vi "Finish.vi"   [LabVIEW 2016]
doc: "This VI is called just before exiting. It is expected to close I/O refnum, save collected data, etc."
uses:
  Climb/Climb Globals.vi
  Drive/Drive Globals.vi
  Intake/Intake Globals.vi
  Rotation/Rotation Globals.vi
  <vilib>/Rock Robotics/WPI/Utilities/WPI_GetSetVariantRefNum.vi
types:
  T1 = typedef "WPI_MotorControlDeviceRef.ctl" = cluster{"DeviceStatus":errorcluster, "Type":T2, "PWM":cluster{"PWM Channel":T3, "DeadBand":T4}, "CAN":cluster{"Device Number":u8, "SetOutput VI Ref":variant, "GetOutput VI Ref":variant, "Enable VI Ref":variant, "Disable VI Ref":variant, "Data":variant}, "Invert":bool}
  T2 = typedef "WPI_MotorControlType.ctl" = enum16{"PWM", "CAN"}
  T3 = typedef "FPGA_DIOPWMChannel.ctl" = enum8{"PWM 0", "PWM 1", "PWM 2", "PWM 3", "PWM 4", "PWM 5", "PWM 6", "PWM 7", "PWM 8", "PWM 9", "PWM MXP 0", "PWM MXP 1", "PWM MXP 2", "PWM MXP 3", "PWM MXP 4", "PWM MXP 5", "PWM MXP 6", "PWM MXP 7", "PWM MXP 8", "PWM MXP 9", "Invalid"}
  T4 = typedef "WPI_PWMDeadband.ctl" = cluster{"Name":string, "maxPositivePwm":i32, "minPositivePwm":i32, "centerPwm":i32, "maxNegativePwm":i32, "minNegativePwm":i32, "angularRange":u16}
  T5 = typedef "WPI_JoystickDevRef.ctl" = cluster{"Device":T6}
  T6 = typedef "WPI_JoystickDeviceEnum.ctl" = enum16{"USB 0", "USB 1", "USB 2", "USB 3", "USB 4", "USB 5"}
  T7 = typedef "WPI_EncoderDevRef.ctl" = cluster{"DevStatus":errorcluster, "EncoderIndex":T8, "CounterIndex":T9, "DistancePerCount":dbl, "Decoding Type":T10}
  T8 = typedef "FPGA_EncoderIdx.ctl" = enum8{"Enc 0", "Enc 1", "Enc 2", "Enc 3", "Enc 4", "Enc 5", "Enc 6", "Enc 7", "Invalid"}
  T9 = typedef "FPGA_CounterCtrSystemIndex.ctl" = enum8{"Ctr 0", "Ctr 1", "Ctr 2", "Ctr 3", "Ctr 4", "Ctr 5", "Ctr 6", "Ctr 7", "Invalid"}
  T10 = typedef "WPI_EncoderType.ctl" = enum16{"1x", "2x", "4x"}
  T11 = typedef "WPI_SwitchDevRef.ctl" = cluster{"DevStatus":errorcluster, "DIO Channel":T12, "CntIndex":T9, "Normally Closed":bool}
  T12 = typedef "FPGA_DIOChannel.ctl" = enum8{"DIO 0", "DIO 1", "DIO 2", "DIO 3", "DIO 4", "DIO 5", "DIO 6", "DIO 7", "DIO 8", "DIO 9", "DIO MXP 0", "DIO MXP 1", "DIO MXP 2", "DIO MXP 3", "DIO MXP 4", "DIO MXP 5", "DIO MXP 6", "DIO MXP 7", "DIO MXP 8", "DIO MXP 9", "DIO MXP 10", "DIO MXP 11", "DIO MXP 12", "DIO MXP 13", "DIO MXP 14", "DIO MXP 15", "SPI Port CS1", "SPI Port CS2", "SPI Port CS3", "SPI Port MISO", "SPI Port MOSI", "Invalid"}
  T13 = typedef "WPI_AnalogChannelDevRef.ctl" = cluster{"DevStatus":errorcluster, "Analog Channel":T14}
  T14 = typedef "FPGA_AIChannel.ctl" = enum8{"AI 0", "AI 1", "AI 2", "AI 3", "AI MXP 0", "AI MXP 1", "AI MXP 2", "AI MXP 3", "Invalid"}
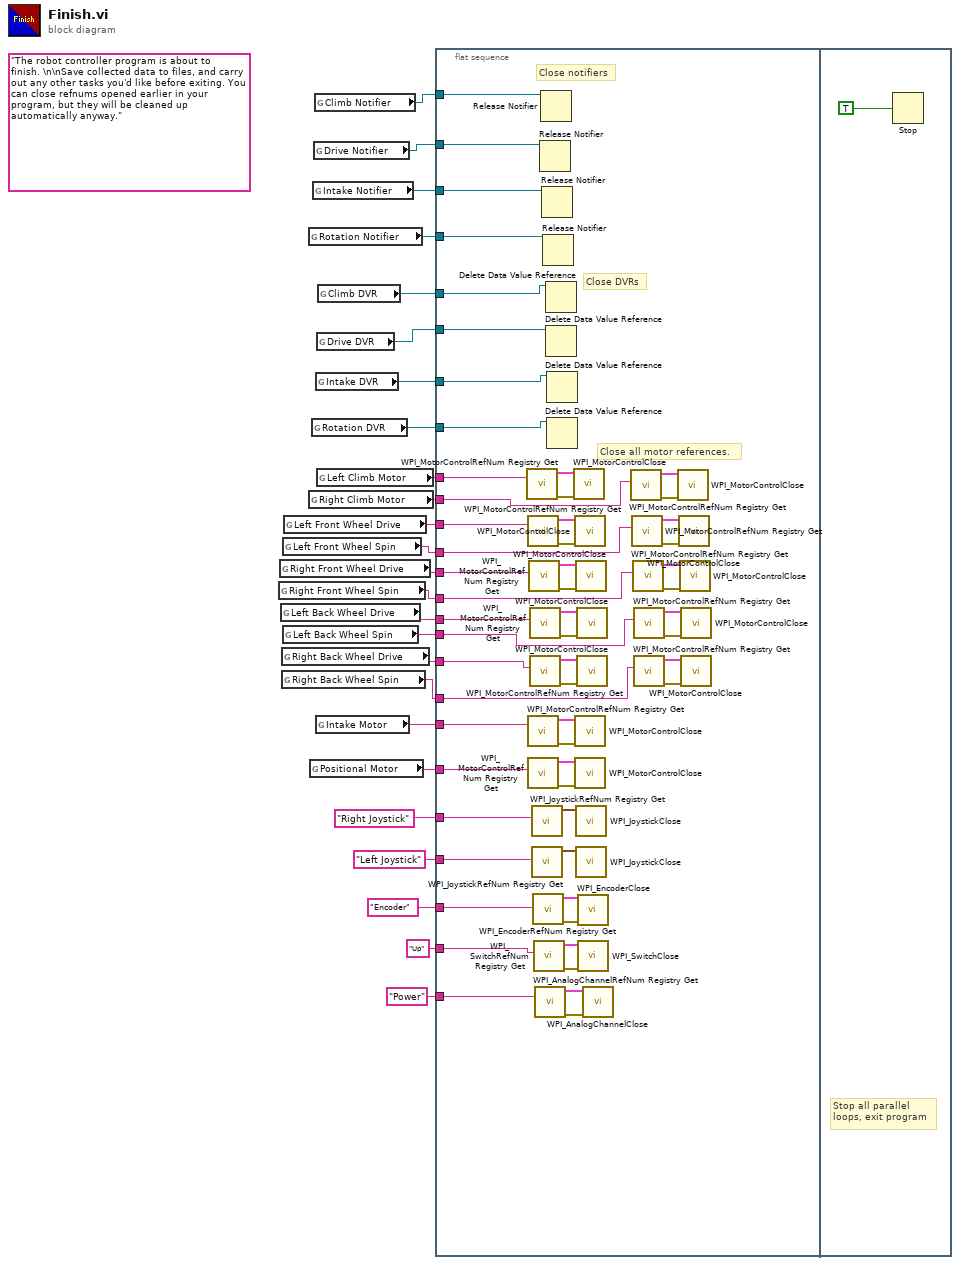
[diagram p0: block diagram]
diagram:
  (unwired) "The robot controller program is about to finish. \n\nSave collected data to files, and carry out any other tasks you'd like before exiting. You can close refnums opened earlier in your program, but they will be cleaned up automatically anyway."
  n1 = global read "Drive Globals.vi" "Right Front Wheel Spin"() -> (w11:string)
  n2 = global read "Drive Globals.vi" "Right Front Wheel Drive"() -> (w15:string)
  n3 = global read "Drive Globals.vi" "Left Back Wheel Drive"() -> (w14:string)
  n4 = global read "Drive Globals.vi" "Right Back Wheel Drive"() -> (w13:string)
  n5 = global read "Drive Globals.vi" "Right Back Wheel Spin"() -> (w9:string)
  n6 = global read "Drive Globals.vi" "Left Front Wheel Spin"() -> (w12:string)
  n7 = global read "Drive Globals.vi" "Left Back Wheel Spin"() -> (w10:string)
  n8 = global read "Drive Globals.vi" "Left Front Wheel Drive"() -> (w16:string)
  n9 = global read "Rotation Globals.vi" "Rotation Notifier"() -> (w22:refnum<notifier>)
  n10 = global read "Climb Globals.vi" "Right Climb Motor"() -> (w8:string)
  n11 = global read "Rotation Globals.vi" "Positional Motor"() -> (w6:string)
  n12 = global read "Rotation Globals.vi" "Rotation DVR"() -> (w18:refnum<data-value>)
  n13 = global read "Intake Globals.vi" "Intake Notifier"() -> (w23:refnum<notifier>)
  n14 = global read "Drive Globals.vi" "Drive Notifier"() -> (w24:refnum<notifier>)
  n15 = global read "Climb Globals.vi" "Climb Notifier"() -> (w25:refnum<notifier>)
  n16 = global read "Intake Globals.vi" "Intake DVR"() -> (w19:refnum<data-value>)
  n17 = global read "Intake Globals.vi" "Intake Motor"() -> (w7:string)
  n18 = global read "Drive Globals.vi" "Drive DVR"() -> (w20:refnum<data-value>)
  n19 = global read "Climb Globals.vi" "Left Climb Motor"() -> (w17:string)
  n20 = global read "Climb Globals.vi" "Climb DVR"() -> (w21:refnum<data-value>)
  n21 = flat-sequence {
    tunnel: w25 -> [w82]
    tunnel: w24 -> [w81]
    tunnel: w23 -> [w80]
    tunnel: w22 -> [w79]
    tunnel: w21 -> [w78]
    tunnel: w20 -> [w77]
    tunnel: w19 -> [w76]
    tunnel: w18 -> [w75]
    tunnel: w17 -> [w74]
    tunnel: w16 -> [w68]
    tunnel: w15 -> [w67]
    tunnel: w14 -> [w63]
    tunnel: w13 -> [w62]
    tunnel: w12 -> [w51]
    tunnel: w11 -> [w50]
    tunnel: w10 -> [w49]
    tunnel: w9 -> [w48]
    tunnel: w8 -> [w45]
    tunnel: w7 -> [w43]
    tunnel: w6 -> [w39]
    tunnel: "Right Joystick" ("refnum name") -> [w36]
    tunnel: "Left Joystick" ("refnum name") -> [w35]
    tunnel: "Encoder" ("refnum name") -> [w32]
    tunnel: "Up" ("refnum name") -> [w31]
    tunnel: "Power" ("refnum name") -> [w28]
    frame #0 {
      # "Close DVRs"
      # "Close all motor references."
      # "Close notifiers"
      n22 = call <vilib>:"WPI_MotorControlRefNum Registry Get.vi"("refnum name"=w74) -> ("error out"=w72:errorcluster, "MotorControlDevRef"=w73:T1)  [unwired: 9 in]
      n23 = call <vilib>:"WPI_MotorControlRefNum Registry Get.vi"("refnum name"=w68) -> ("error out"=w71:errorcluster, "MotorControlDevRef"=w65:T1)  [unwired: 9 in]
      n24 = call <vilib>:"WPI_MotorControlRefNum Registry Get.vi"("refnum name"=w43) -> ("error out"=w44:errorcluster, "MotorControlDevRef"=w42:T1)  [unwired: 9 in]
      n25 = call <vilib>:"WPI_MotorControlRefNum Registry Get.vi"("refnum name"=w39) -> ("error out"=w41:errorcluster, "MotorControlDevRef"=w40:T1)  [unwired: 9 in]
      n26 = call <vilib>:"WPI_MotorControlRefNum Registry Get.vi"("refnum name"=w67) -> ("error out"=w69:errorcluster, "MotorControlDevRef"=w66:T1)  [unwired: 9 in]
      n27 = call <vilib>:"WPI_MotorControlRefNum Registry Get.vi"("refnum name"=w63) -> ("error out"=w70:errorcluster, "MotorControlDevRef"=w60:T1)  [unwired: 9 in]
      n28 = call <vilib>:"WPI_MotorControlRefNum Registry Get.vi"("refnum name"=w62) -> ("error out"=w64:errorcluster, "MotorControlDevRef"=w61:T1)  [unwired: 9 in]
      n29 = call <vilib>:"WPI_JoystickRefNum Registry Get.vi"("refnum name"=w36) -> ("JoystickDevRef"=w38:T5)  [unwired: 9 in, 1 out]
      n30 = call <vilib>:"WPI_JoystickRefNum Registry Get.vi"("refnum name"=w35) -> ("JoystickDevRef"=w37:T5)  [unwired: 9 in, 1 out]
      n31 = call <vilib>:"WPI_EncoderRefNum Registry Get.vi"("refnum name"=w32) -> ("error out"=w26:errorcluster, "EncoderDevRef"=w27:T7)  [unwired: 9 in]
      n32 = call <vilib>:"WPI_SwitchRefNum Registry Get.vi"("refnum name"=w31) -> ("error out"=w34:errorcluster, "SwitchDevRef"=w33:T11)  [unwired: 9 in]
      n33 = call <vilib>:"WPI_AnalogChannelRefNum Registry Get.vi"("refnum name"=w28) -> ("error out"=w30:errorcluster, "AIDeviceRef"=w29:T13)  [unwired: 9 in]
      n34 = Release Notifier(notifier=w81) -> ()  [unwired: 2 in, 3 out]
      n35 = Release Notifier(notifier=w82) -> ()  [unwired: 2 in, 3 out]
      n36 = Release Notifier(notifier=w80) -> ()  [unwired: 2 in, 3 out]
      n37 = Release Notifier(notifier=w79) -> ()  [unwired: 2 in, 3 out]
      n38 = Delete Data Value Reference(data value reference=w78) -> ()  [unwired: 1 in, 2 out]
      n39 = Delete Data Value Reference(data value reference=w77) -> ()  [unwired: 1 in, 2 out]
      n40 = Delete Data Value Reference(data value reference=w76) -> ()  [unwired: 1 in, 2 out]
      n41 = Delete Data Value Reference(data value reference=w75) -> ()  [unwired: 1 in, 2 out]
      n42 = call <vilib>:"WPI_MotorControlClose.vi"("error in"=w72, "MotorControlDevRef"=w73) -> ()  [unwired: 9 in, 1 out]
      n43 = call <vilib>:"WPI_MotorControlClose.vi"("error in"=w71, "MotorControlDevRef"=w65) -> ()  [unwired: 9 in, 1 out]
      n44 = call <vilib>:"WPI_MotorControlClose.vi"("error in"=w44, "MotorControlDevRef"=w42) -> ()  [unwired: 9 in, 1 out]
      n45 = call <vilib>:"WPI_MotorControlClose.vi"("error in"=w41, "MotorControlDevRef"=w40) -> ()  [unwired: 9 in, 1 out]
      n46 = call <vilib>:"WPI_MotorControlClose.vi"("error in"=w69, "MotorControlDevRef"=w66) -> ()  [unwired: 9 in, 1 out]
      n47 = call <vilib>:"WPI_JoystickClose.vi"("JoystickDevRef"=w38) -> ()  [unwired: 11 in]
      n48 = call <vilib>:"WPI_JoystickClose.vi"("JoystickDevRef"=w37) -> ()  [unwired: 11 in]
      n49 = call <vilib>:"WPI_MotorControlClose.vi"("error in"=w70, "MotorControlDevRef"=w60) -> ()  [unwired: 9 in, 1 out]
      n50 = call <vilib>:"WPI_MotorControlClose.vi"("error in"=w64, "MotorControlDevRef"=w61) -> ()  [unwired: 9 in, 1 out]
      n51 = call <vilib>:"WPI_EncoderClose.vi"("error in (no error)"=w26, "EncoderDevRef"=w27) -> ()  [unwired: 9 in, 1 out]
      n52 = call <vilib>:"WPI_SwitchClose.vi"("error in (no error)"=w34, "SwitchDevRef"=w33) -> ()  [unwired: 9 in, 1 out]
      n53 = call <vilib>:"WPI_AnalogChannelClose.vi"("error in (no error)"=w30, "AIDeviceRef"=w29) -> ()  [unwired: 9 in, 1 out]
      n54 = call <vilib>:"WPI_MotorControlRefNum Registry Get.vi"("refnum name"=w45) -> ("error out"=w46:errorcluster, "MotorControlDevRef"=w47:T1)  [unwired: 9 in]
      n55 = call <vilib>:"WPI_MotorControlRefNum Registry Get.vi"("refnum name"=w51) -> ("error out"=w59:errorcluster, "MotorControlDevRef"=w55:T1)  [unwired: 9 in]
      n56 = call <vilib>:"WPI_MotorControlRefNum Registry Get.vi"("refnum name"=w50) -> ("error out"=w57:errorcluster, "MotorControlDevRef"=w56:T1)  [unwired: 9 in]
      n57 = call <vilib>:"WPI_MotorControlRefNum Registry Get.vi"("refnum name"=w49) -> ("error out"=w58:errorcluster, "MotorControlDevRef"=w52:T1)  [unwired: 9 in]
      n58 = call <vilib>:"WPI_MotorControlRefNum Registry Get.vi"("refnum name"=w48) -> ("error out"=w54:errorcluster, "MotorControlDevRef"=w53:T1)  [unwired: 9 in]
      n59 = call <vilib>:"WPI_MotorControlClose.vi"("error in"=w46, "MotorControlDevRef"=w47) -> ()  [unwired: 9 in, 1 out]
      n60 = call <vilib>:"WPI_MotorControlClose.vi"("error in"=w59, "MotorControlDevRef"=w55) -> ()  [unwired: 9 in, 1 out]
      n61 = call <vilib>:"WPI_MotorControlClose.vi"("error in"=w57, "MotorControlDevRef"=w56) -> ()  [unwired: 9 in, 1 out]
      n62 = call <vilib>:"WPI_MotorControlClose.vi"("error in"=w58, "MotorControlDevRef"=w52) -> ()  [unwired: 9 in, 1 out]
      n63 = call <vilib>:"WPI_MotorControlClose.vi"("error in"=w54, "MotorControlDevRef"=w53) -> ()  [unwired: 9 in, 1 out]
    }
    frame #1 {
      # "Stop all parallel\nloops, exit program"
      n64 = Stop(stop? (T)=TRUE ("Quit")) -> ()
    }
  }
